vi "Modulation Table Set Row.vi"(7 "Row":i8=1 min=1 max=20 step=1, 8 "error in (no error)":errorcluster, 9 "Modulation Factor":dbl format="%.3f", 10 "Modulation Voltage":dbl format="%.3f", 11 "VISA session in":refnum<visa-resource-name>) -> (0 "error out":errorcluster, 3 "VISA session out":refnum<visa-resource-name>)   [LabVIEW 2011, in "Magna PSU.lvlib"]
uses:
  Magna PSU.lvlib
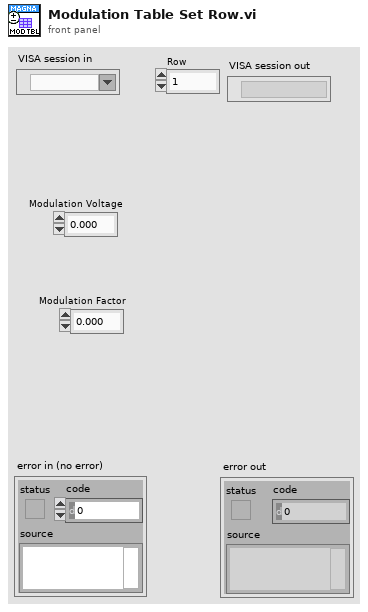
[diagram p1: front panel]
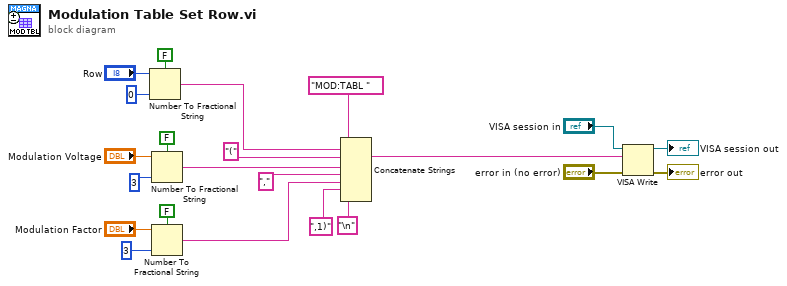
[diagram p0: block diagram]
diagram:
  n1 = Number To Fractional String(use system decimal point (T)=FALSE, number="Row", precision (6)=0) -> (F-format string=w7:string)  [unwired: 1 in]
  n2 = Number To Fractional String(use system decimal point (T)=FALSE, number="Modulation Voltage", precision (6)=3) -> (F-format string=w6:string)  [unwired: 1 in]
  n3 = Number To Fractional String(use system decimal point (T)=FALSE, number="Modulation Factor", precision (6)=3) -> (F-format string=w5:string)  [unwired: 1 in]
  n4 = Concatenate Strings("MOD:TABL ", w7, "(", w6, ",", w5, ",1)", "\n") -> (w4:string)
  n5 = VISA Write(VISA resource name="VISA session in", write buffer=w4, error in (no error)="error in (no error)") -> (VISA resource name out=→"VISA session out":refnum<visa-resource-name>, error out=→"error out":errorcluster)  [unwired: 1 out]
